vi "Divide.vi"(8 "Y":dbl, 11 "X":dbl) -> (3 "X/Y":dbl)   [LabVIEW 2019, in "Simple Math Toolkit.lvlib"]
uses:
  Simple Math Toolkit.lvlib
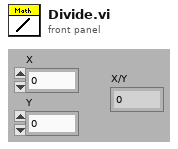
[diagram p1: front panel]
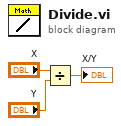
[diagram p0: block diagram]
diagram:
  n1 = Divide(x="X", y="Y") -> (x/y=→"X/Y":dbl)
